vi "Database-Disconnect.vi"(8 "error in":errorcluster, 11 "Idx":i32) -> (0 "error out":errorcluster)   [LabVIEW 2016]
uses:
  Database.Action.ctl
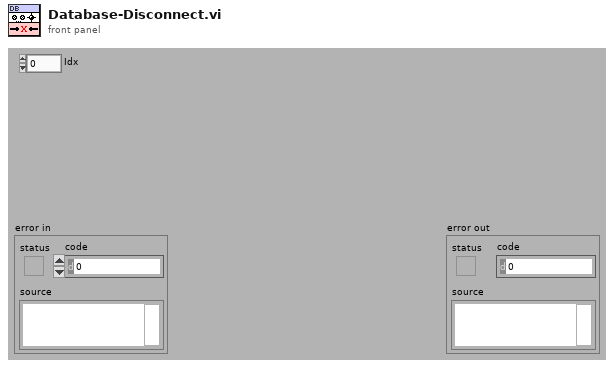
[diagram p1: front panel]
types:
  T1 = typedef "Database.Action.ctl" = enum32{"idle", "constructor", "destructor", "--- DB ---", "Setup", "Disconnect", "Connect", "GetThisStatus"}
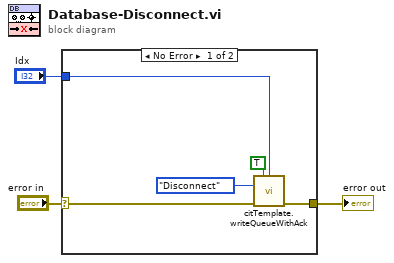
[diagram p0: block diagram]
diagram:
  n1 = case shown="No Error" "error in" {
    selector: "error in" -> [w7 w9]
    tunnel: [w8 w9] -> w2
    tunnel: "Idx" -> [w4 _]
    frame No Error {
      n2 = call "citTemplate.writeQueueWithAck.vi"("High priority (F)"=TRUE, "instance (0)"=w4, "event in"=Database.Action."Disconnect" ("Action"), "error in (no error)"=w7) -> ("error out"=w8:errorcluster)  [unwired: 9 in, 2 out]
    }
    frame Error {
    }
  }
  "error out" <- w2
